vi "Is Supported Cluster.vi"(11 "variant":variant) -> (2 "message_type":string, 3 "supported?":bool)   [LabVIEW 2020, in "MeasurementLink Measurement Server.lvlib"]
uses:
  MeasurementLink Measurement Server.lvlib
  gRPC/Generated APIs/ni/protobuf/types/RPC Messages/ni_protobuf_types_DoubleXYData.ctl
  88eec10a-a3aa-4f92-886f-65a0ec068e4c.vi
  <vilib>/Comparison/Equal/Equal Functor/Equal Functor.lvclass
  <vilib>/Utility/Data Type/NI_Data Type.lvlib
  gRPC/Generated APIs/ni/protobuf/types/ni.protobuf.types.lvlib
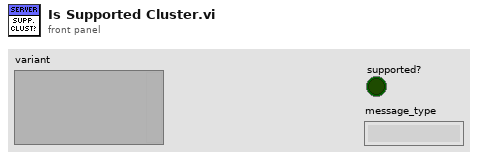
[diagram p1: front panel]
types:
  T1 = typedef "ni.protobuf.types.lvlib/ni_protobuf_types_DoubleXYData.ctl" = cluster{"x_data":dbl[], "y_data":dbl[]}
  T2 = typedef "NI_Data Type.lvlib/Type Definition Info.ctl" = cluster{"Name":string, "Timestamp":u32}
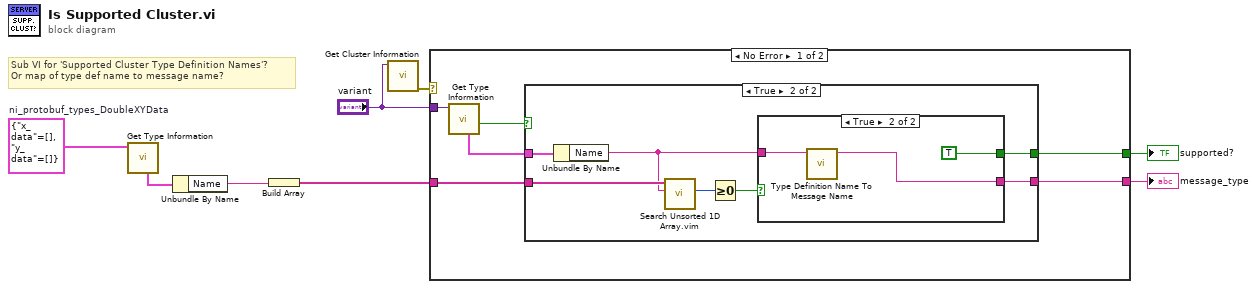
[diagram p0: block diagram]
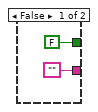
[diagram p2: hidden frame]
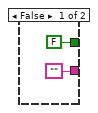
[diagram p3: hidden frame]
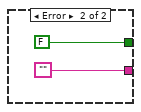
[diagram p4: hidden frame]
diagram:
  w4 = T1 {"x_data"=[], "y_data"=[]}  # ni_protobuf_types_DoubleXYData
  # "Sub VI for 'Supported Cluster Type Definition Names'?\nOr map of type def name to message name?"
  n1 = call <vilib>:"Get Type Information.vi"("variant"=w4) -> ("type definition info"=w3:T2)  [unwired: 6 in, 4 out]
  n2 = Unbundle By Name(w3) -> ("Name"=w2:string)
  n3 = Build Array(w2) -> (w1:string[])
  n4 = call <vilib>:"Get Cluster Information.vi"("variant"="variant") -> ("error out"=w7:errorcluster)  [unwired: 9 in, 1 out]
  n5 = case shown="No Error" w7 {
    tunnel: [w11 FALSE] -> w8
    tunnel: [w10 ""] -> w6
    tunnel: "variant" -> [w14 _]
    tunnel: w1 -> [w9 _]
    frame No Error {
      n6 = call <vilib>:"Get Type Information.vi"("variant"=w14) -> ("type definition"=w12:bool, "type definition info"=w13:T2)  [unwired: 6 in, 3 out]
      n7 = case shown="True" w12 {
        tunnel: w13 -> [_ w23]
        tunnel: [FALSE w22] -> w11
        tunnel: ["" w21] -> w10
        tunnel: w9 -> [_ w20]
        frame False {
        }
        frame True {
          n8 = Unbundle By Name(w23) -> ("Name"=w17:string)
          n9 = call "Search Unsorted 1D Array.vim"("element"=w17, "unsorted 1D array"=w20) -> ("index of element"=w19:i32)  [unwired: 9 in]
          n10 = Greater Or Equal To 0?(x=w19) -> (x >= 0?=w18:bool)
          n11 = case shown="True" w18 {
            tunnel: [FALSE TRUE] -> w22
            tunnel: ["" w26] -> w21
            tunnel: w17 -> [_ w27]
            frame False {
            }
            frame True {
              n12 = call "Type Definition Name To Message Name.vi"("type definition name"=w27) -> ("message name"=w26:string)  [unwired: 10 in]
            }
          }
        }
      }
    }
    frame Error {
    }
  }
  "supported?" <- w8
  "message_type" <- w6
